vi "Read Output Array.vi"(8 "error in (no error)":errorcluster, 11 "DtoA in":refnum<class "External Clock.lvclass">) -> (0 "error out":errorcluster, 2 "Output Array":u16[](array[numeric]), 3 "DtoA out":refnum<class "External Clock.lvclass">)   [LabVIEW 2014, in "External Clock.lvclass"]
uses:
  External Clock.lvclass
  External Clock.lvclass/External Clock.ctl
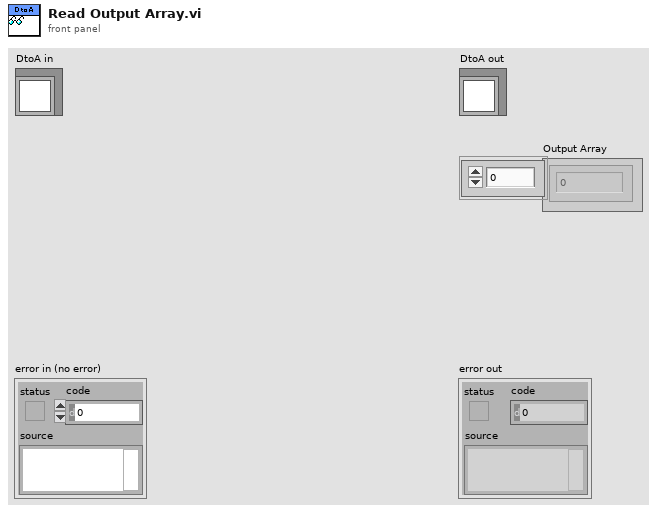
[diagram p1: front panel]
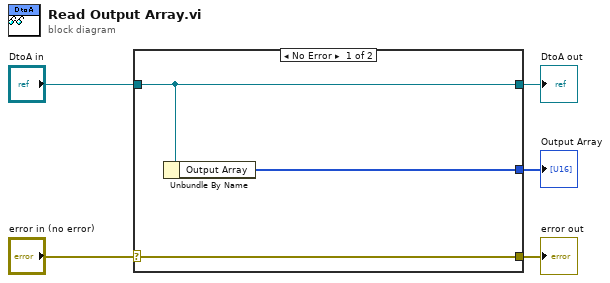
[diagram p0: block diagram]
diagram:
  n1 = case shown="No Error" "error in (no error)" {
    selector: "error in (no error)" -> [w8 w9]
    tunnel: [w8 w9] -> w4
    tunnel: [w7 w10] -> w2
    tunnel: "DtoA in" -> [w7 w10]
    tunnel: [w6 _] -> w1
    frame No Error {
      n2 = Unbundle By Name(w7) -> ("Output Array"=w6:u16[])
    }
    frame Error {
    }
  }
  "error out" <- w4
  "DtoA out" <- w2
  "Output Array" <- w1
